vi "Variables globales outil isospi sans MCU.vi"() -> ()   [LabVIEW 2019]
panel:
  out "CTNcoeffC":dbl
  out "CTNcoeffB":dbl
  out "CTNcoeffA":dbl
  out "NumberofCTNsperCMU":u32
  out "NumberofCellsperCMU":u32
  out "NumberofCMUs":u32
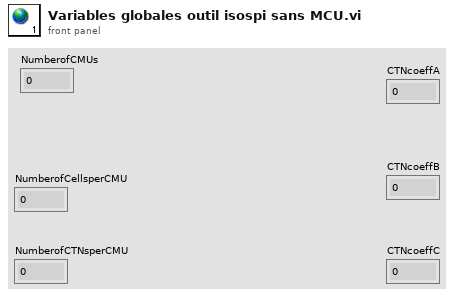
[diagram p1: front panel]
diagram:
